vi "Main.vi"() -> ()   [LabVIEW 2013]
panel:
  in  "Attachment Settings":T1={"Attachment Size"=1.0, "Resize Type"=enum."Size"} {"Attachment Size" scale=0.0..1.0 scale format="%#_2f"}
  out "Last Time Checked":timestamp format="%<%I:%M:%S %p\n%x>T"
  in  "Send Images?":bool
  in  "Log Information?":bool=TRUE
  in  "Log File Path":path
  out "Number of Files in Directory":i32
  in  "Load Contacts":bool
  in  "Save Contacts":bool
  in  "Email Password":string="apatite2Z"
  in  "Email Username":string="raymond.apatite@gmail.com"
  in  "SMTP Server":string="smtp.gmail.com"
  in  "Extension":string
  in  "Contacts":T2(array[cluster])=[{"Name"="Margaret Donelick", "Phone Number"="2085961690", "Wireless Carrier"=enum."AT&T", "Email Address"="donelick@apatite.com", "Has Texting?"=TRUE}, {"Name"="Ray Donelick", "Phone Number"="2085961423", "Wireless Carrier"=enum."AT&T", "Email Address"="donelick@apatite.com", "Has Texting?"=FALSE}, {"Name"="Andrew Donelick", "Phone Number"="2085969583", "Wireless Carrier"=enum."AT&T", "Email Address"="adonelick@g.hmc.edu", "Has Texting?"=FALSE}, {"Name"="Helen Donelick", "Phone Number"="2085965021", "Wireless Carrier"=enum."AT&T", "Email Address"="done5409@pacificu.edu", "Has Texting?"=TRUE}]
  in  "Message Body":string="The is a possible problem."
  in  "Message Subject":string="Check the Laser!"
  in  "Monitor Folder?":bool
  in  "Person to Contact":u16(ring) items=["Margaret Donelick", "Ray Donelick", "Andrew Donelick", "Helen Donelick"]
  in  "Action on Error":T3(ring)
  in  "Check Time (minutes)":i32=60
  in  "Image Folder Directory":path
  out "error out":errorcluster
  in  "error in (no error)":errorcluster
  in  "Stop":bool
  # "Monitoring Settings"
  # "Attachment Settings"
  # "Contact Information"
  # "Message Settings"
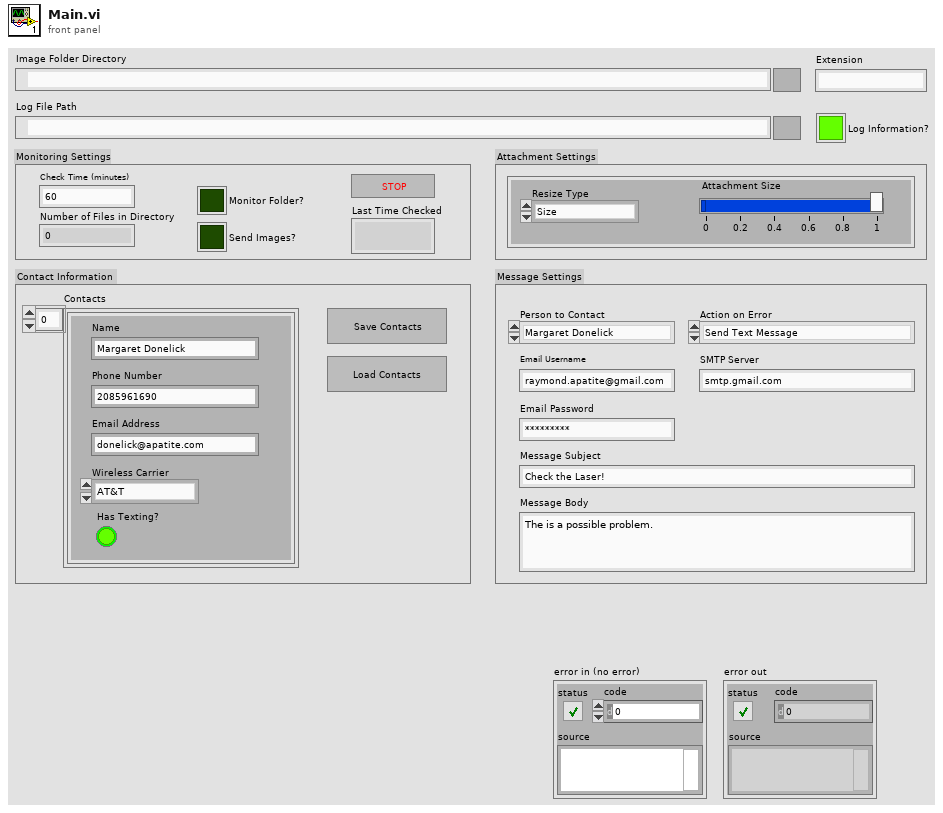
[diagram p1: front panel]
types:
  T1 = cluster{"Attachment Size":dbl, "Resize Type":enum16{"Size", "Resolution"}}
  T2 = cluster{"Name":string, "Phone Number":string, "Wireless Carrier":enum16{"T-Mobile", "AT&T", "Verizon", "Sprint"}, "Email Address":string, "Has Texting?":bool}[]
  T3 = enum16{"Send Text Message", "Send Email", "Send Text Message & Email"}
  T4 = enum16{"open", "replace", "create", "open or create", "replace or create", "replace or create with confirmation"}
  T5 = cluster{"Name":string, "Phone Number":string, "Wireless Carrier":enum16{"T-Mobile", "AT&T", "Verizon", "Sprint"}, "Email Address":string, "Has Texting?":bool}
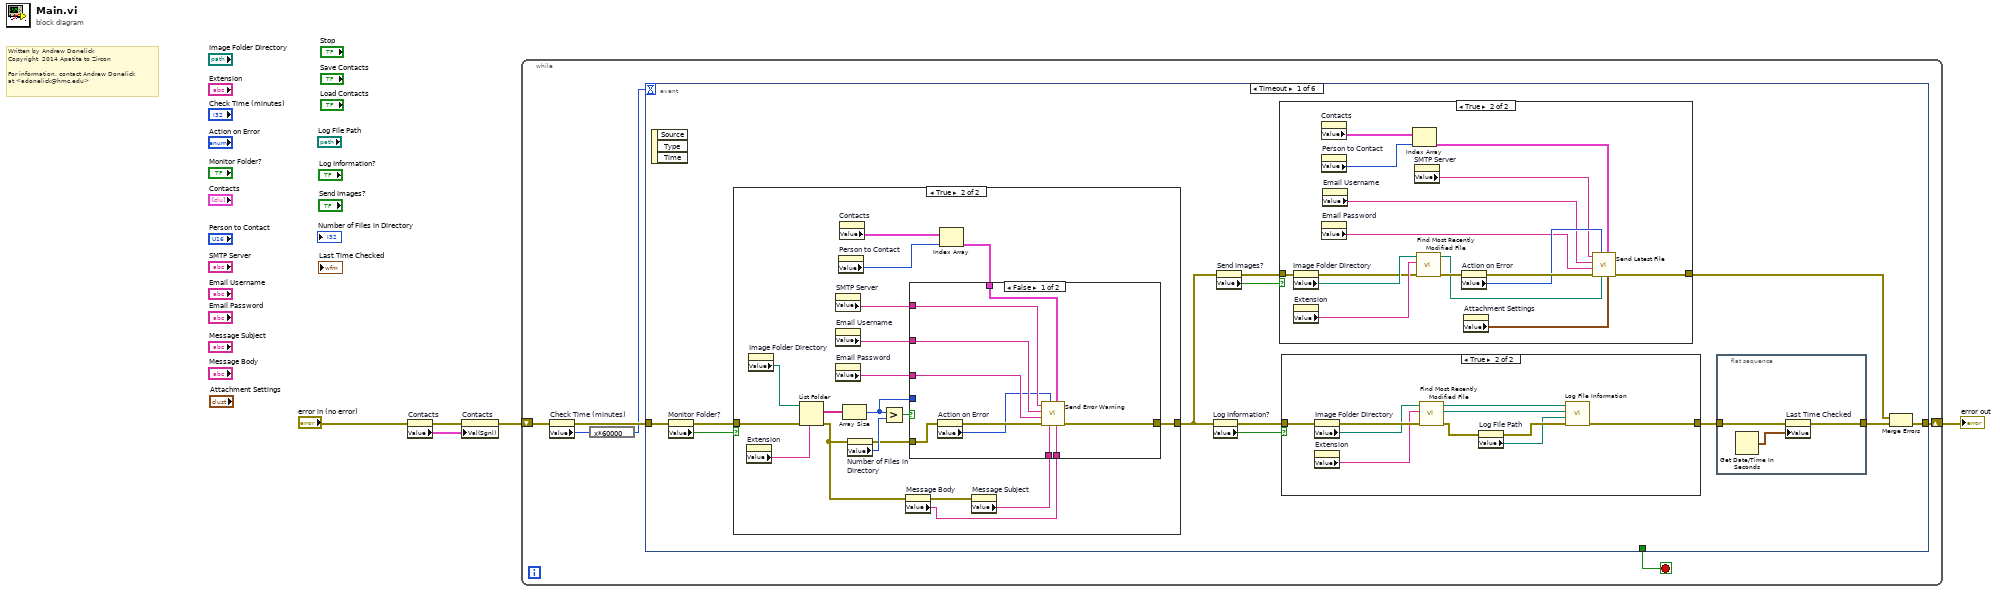
[diagram p0: block diagram]
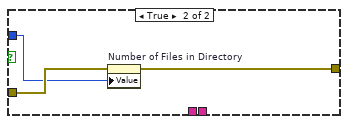
[diagram p5: hidden frame]
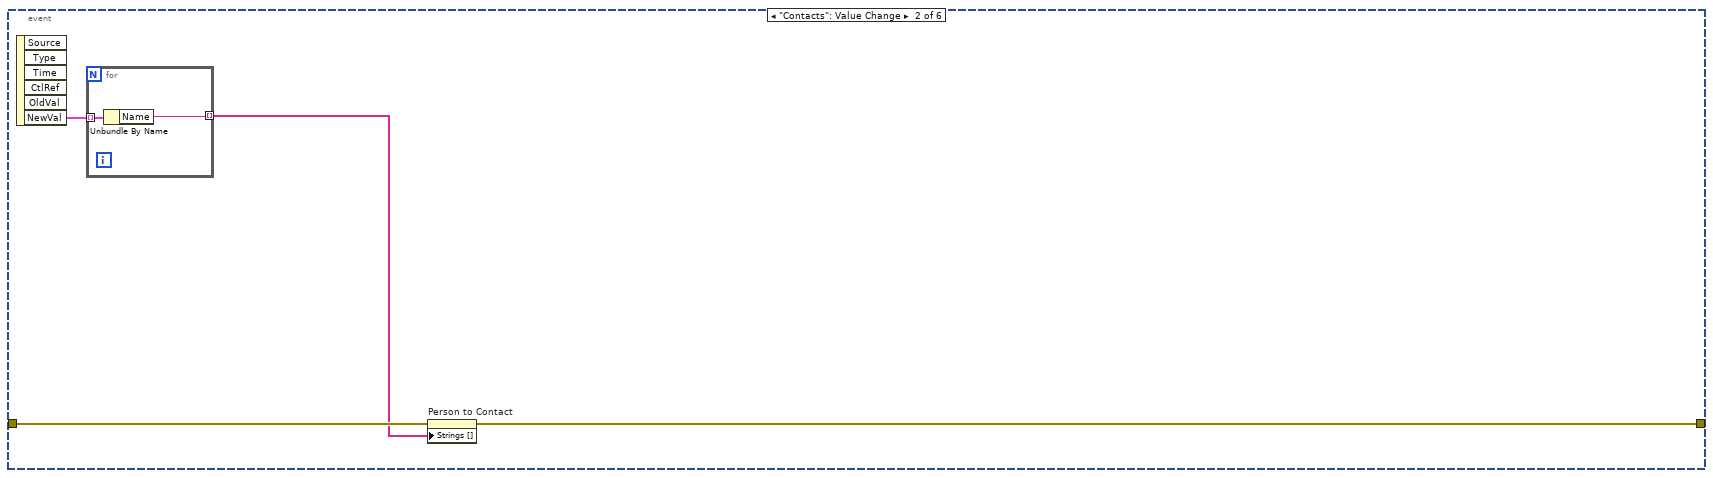
[diagram p6: hidden frame]
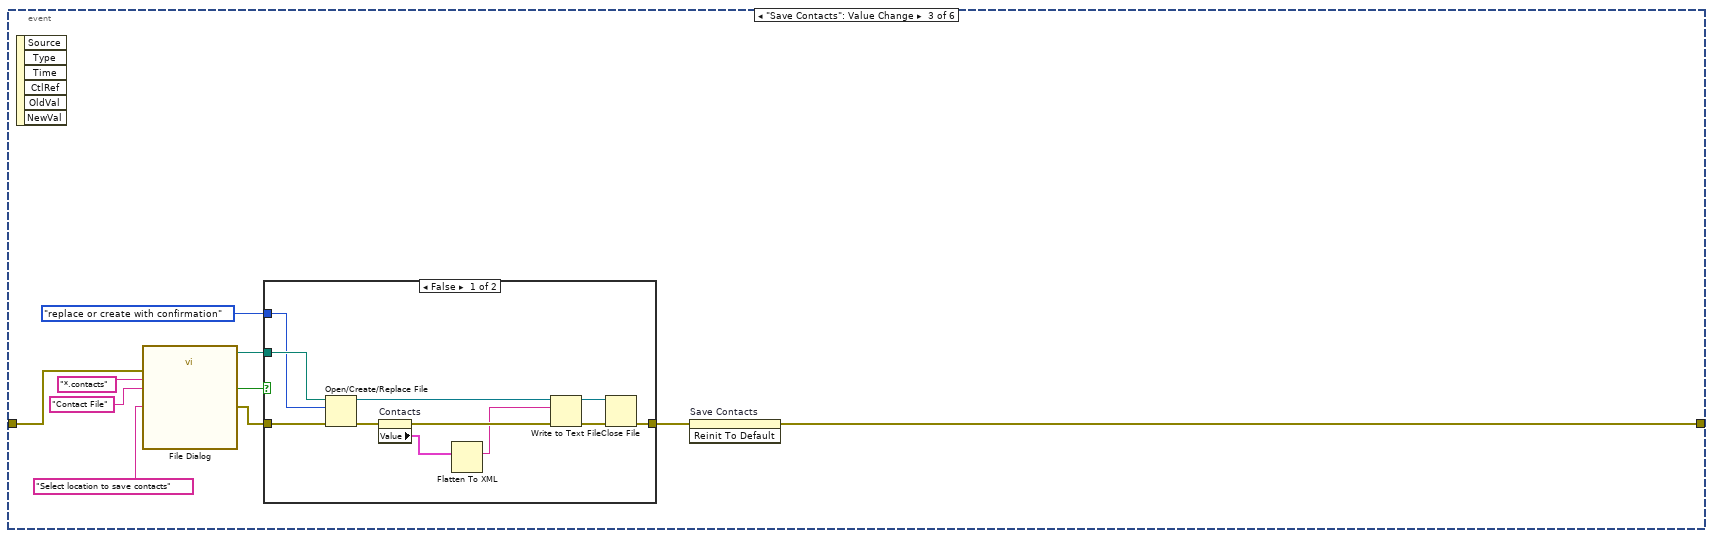
[diagram p7: hidden frame]
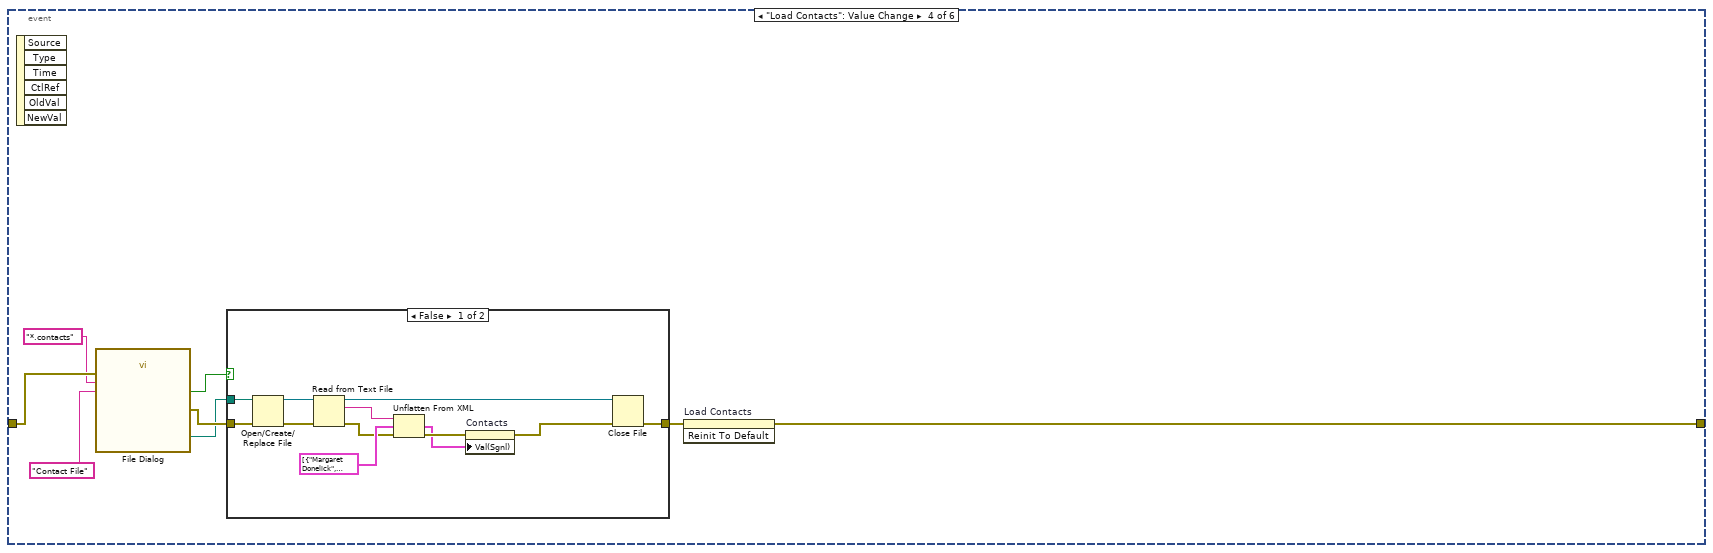
[diagram p9: hidden frame]
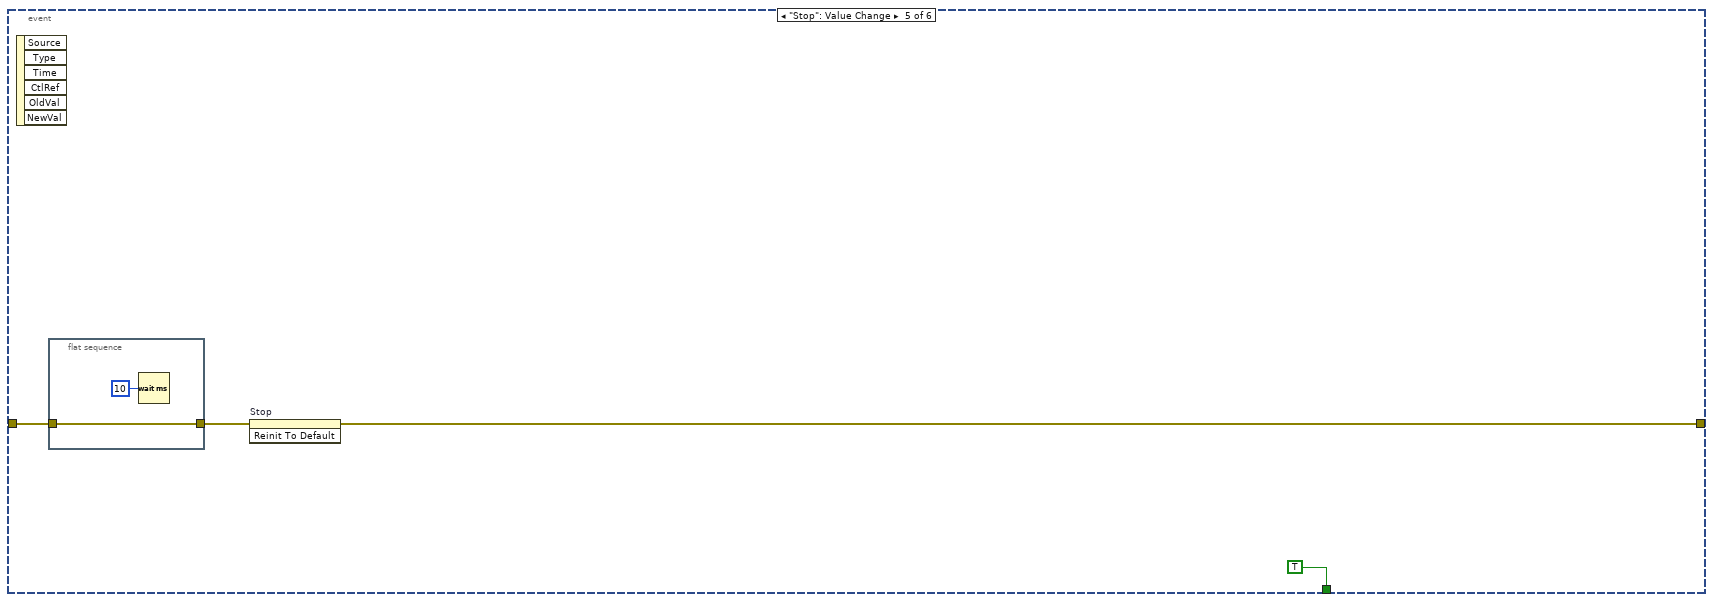
[diagram p11: hidden frame]
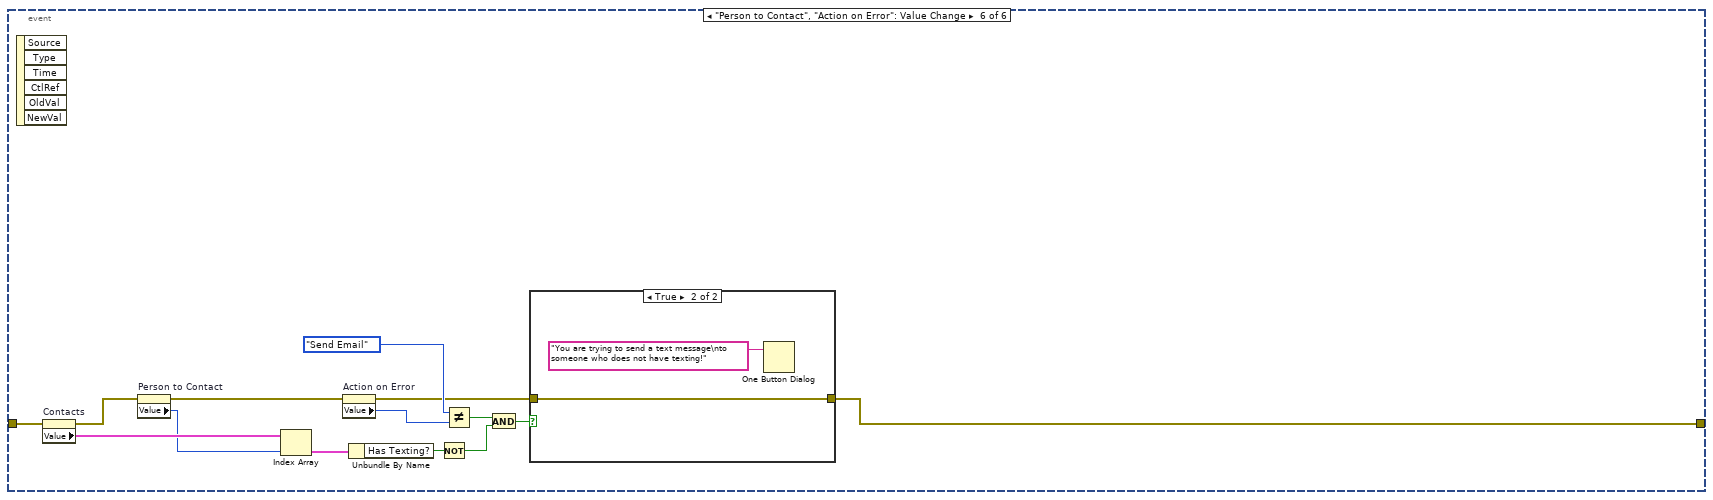
[diagram p12: hidden frame]
diagram:
  # "Written by Andrew Donelick\nCopyright  2014 Apatite to Zircon\n\nFor information, contact Andrew Donelick\nat <adonelick@hmc.edu>"
  n1 = property on="Contacts" class="Arr (strict)"(error in="error in (no error)") -> (error out=w4:errorcluster, "Value"=w3:T2)  [unwired: 1 in, 1 out]
  n2 = property on="Contacts" class="Arr (strict)"(error in=w4, "Val(Sgnl)"=w3) -> (error out=w1:errorcluster)  [unwired: 1 in, 1 out]
  n3 = while {
    shift-right: [w10] -> w5
    shift-left: w1 -> [w8]
    stop <- w11 stop-if-true
    n4 = property on="Check Time (minutes)" class="DigNum (strict)"(error in=w8) -> (error out=w7:errorcluster, "Value"=w9:i32)  [unwired: 1 in, 1 out]
    n5 = expression code="x*60000"(w9) -> (w6:i32)
    n6 = event shown="[0] Timeout" {
      selector: _ -> [_ _ _ _ _ _]
      dyn-events: _ -> [_ _ _ _ _ _]
      timeout: w6 -> [_ _ _ _ _ _]
      tunnel: [_ _ _ _ TRUE _] -> w11
      tunnel: w7 -> [w23 w90 w101 w122 w139 w156]
      tunnel: [w15 w89 w102 w123 w137 w146] -> w10
      event Timeout {
        n7 = event-data() -> ()  [unwired: 1 in, 3 out]
        n8 = property on="Monitor Folder?" class="Bool (strict)"(error in=w23) -> (error out=w22:errorcluster, "Value"=w21:bool)  [unwired: 1 in, 1 out]
        n9 = case shown="True" w21 {
          tunnel: w22 -> [w55 w73]
          tunnel: [w55 w70] -> w16
          frame False {
          }
          frame True {
            n10 = property on="Extension" class="Str"() -> ("Value"=w72:string)  [unwired: 2 in, 2 out]
            n11 = property on="Image Folder Directory" class="Path"() -> ("Value"=w74:path)  [unwired: 2 in, 2 out]
            n12 = List Folder(path=w74, pattern=w72, error in=w73) -> (filenames=w71:string[], error out=w61:errorcluster)  [unwired: 1 in, 2 out]
            n13 = property on="SMTP Server" class="Str"() -> ("Value"=w60:string)  [unwired: 2 in, 2 out]
            n14 = property on="Email Username" class="Str"() -> ("Value"=w59:string)  [unwired: 2 in, 2 out]
            n15 = property on="Email Password" class="Str"() -> ("Value"=w58:string)  [unwired: 2 in, 2 out]
            n16 = property on="Person to Contact" class="Ring (strict)"() -> ("Value"=w65:u16)  [unwired: 2 in, 2 out]
            n17 = property on="Contacts" class="Arr (strict)"() -> ("Value"=w66:T2)  [unwired: 2 in, 2 out]
            n18 = Array Size(array=w71) -> (size(s)=w57:i32)
            n19 = property on="Number of Files in Directory" class="DigNum (strict)"(error in=w61) -> (error out=w67:errorcluster, "Value"=w69:i32)  [unwired: 1 in, 1 out]
            n20 = Greater?(x=w57, y=w69) -> (0:w68:bool)
            n21 = property on="Message Body" class="Str"(error in=w61) -> (error out=w64:errorcluster, "Value"=w62:string)  [unwired: 1 in, 1 out]
            n22 = Index Array(array=w66, index=w65) -> (element=w56:T5)
            n23 = property on="Message Subject" class="Str"(error in=w64) -> ("Value"=w63:string)  [unwired: 1 in, 2 out]
            n24 = case shown="False" w68 {
              tunnel: [w82 w85] -> w70
              tunnel: w67 -> [w84 w87]
              tunnel: w63 -> [w77 _]
              tunnel: w62 -> [w76 _]
              tunnel: w60 -> [w81 _]
              tunnel: w59 -> [w80 _]
              tunnel: w58 -> [w79 _]
              tunnel: w57 -> [_ w86]
              tunnel: w56 -> [w78 _]
              frame False {
                n25 = property on="Action on Error" class="Enum (strict)"(error in=w84) -> (error out=w83:errorcluster, "Value"=w75:T3)  [unwired: 1 in, 1 out]
                n26 = call "Send Error Warning.vi"("Message Body"=w76, "Contact"=w78, "Message Subject"=w77, "Action on Error"=w75, "error in"=w83, "Email Password"=w79, "Email Username"=w80, "SMTP Server"=w81) -> ("error out"=w82:errorcluster)  [unwired: 3 in]
              }
              frame True {
                n27 = property on="Number of Files in Directory" class="DigNum (strict)"(error in=w87, "Value"=w86) -> (error out=w85:errorcluster)  [unwired: 1 in, 1 out]
              }
            }
          }
        }
        n28 = property on="Log Information?" class="Bool (strict)"(error in=w16) -> (error out=w20:errorcluster, "Value"=w19:bool)  [unwired: 1 in, 1 out]
        n29 = property on="Send Images?" class="Bool (strict)"(error in=w16) -> (error out=w17:errorcluster, "Value"=w18:bool)  [unwired: 1 in, 1 out]
        n30 = case shown="True" w18 {
          tunnel: w17 -> [w27 w31]
          tunnel: [w27 w29] -> w14
          frame False {
          }
          frame True {
            n31 = property on="Image Folder Directory" class="Path"(error in=w31) -> (error out=w32:errorcluster, "Value"=w43:path)  [unwired: 1 in, 1 out]
            n32 = property on="Extension" class="Str"() -> ("Value"=w42:string)  [unwired: 2 in, 2 out]
            n33 = property on="Contacts" class="Arr (strict)"() -> ("Value"=w35:T2)  [unwired: 2 in, 2 out]
            n34 = property on="Person to Contact" class="Ring (strict)"() -> ("Value"=w34:u16)  [unwired: 2 in, 2 out]
            n35 = property on="Email Password" class="Str"() -> ("Value"=w33:string)  [unwired: 2 in, 2 out]
            n36 = property on="Email Username" class="Str"() -> ("Value"=w30:string)  [unwired: 2 in, 2 out]
            n37 = Index Array(array=w35, index=w34) -> (element=w38:T5)
            n38 = property on="SMTP Server" class="Str"() -> ("Value"=w37:string)  [unwired: 2 in, 2 out]
            n39 = call "Find Most Recently Modified File.vi"("error in (no error)"=w32, "Pattern"=w42, "Directory"=w43) -> ("error out"=w41:errorcluster, "Most Recent File Path"=w36:path)  [unwired: 5 in, 1 out]
            n40 = property on="Action on Error" class="Enum (strict)"(error in=w41) -> (error out=w40:errorcluster, "Value"=w39:T3)  [unwired: 1 in, 1 out]
            n41 = property on="Attachment Settings" class="Clust (strict)"() -> ("Value"=w28:T1)  [unwired: 2 in, 2 out]
            n42 = call "Send Latest File.vi"("Attachment Settings"=w28, "Contact"=w38, "Most Recently Modified Image Path"=w36, "Action on Error"=w39, "error in"=w40, "Email Password"=w33, "Email Username"=w30, "SMTP Server"=w37) -> ("error out"=w29:errorcluster)  [unwired: 3 in]
          }
        }
        n43 = case shown="True" w19 {
          tunnel: [w44 w51] -> w13
          tunnel: w20 -> [w44 w45]
          frame False {
          }
          frame True {
            n44 = property on="Image Folder Directory" class="Path"(error in=w45) -> (error out=w54:errorcluster, "Value"=w53:path)  [unwired: 1 in, 1 out]
            n45 = property on="Extension" class="Str"() -> ("Value"=w52:string)  [unwired: 2 in, 2 out]
            n46 = call "Find Most Recently Modified File.vi"("error in (no error)"=w54, "Pattern"=w52, "Directory"=w53) -> ("error out"=w48:errorcluster, "2nd Most Recent File Path"=w49:path, "Most Recent File Path"=w50:path)  [unwired: 5 in]
            n47 = property on="Log File Path" class="Path"(error in=w48) -> (error out=w47:errorcluster, "Value"=w46:path)  [unwired: 1 in, 1 out]
            n48 = call "Log File Information.vi"("error in (no error)"=w47, "Log File Path"=w46, "2nd Most Recent File Path"=w49, "Most Recent File Path"=w50) -> ("error out"=w51:errorcluster)  [unwired: 7 in]
          }
        }
        n49 = flat-sequence {
          tunnel: w13 -> [w26]
          tunnel: [w25] -> w12
          frame #0 {
            n50 = Get Date/Time In Seconds() -> (seconds since 1Jan1904=w24:timestamp)
            n51 = property on="Last Time Checked" class="AbsTime (strict)"(error in=w26, "Value"=w24) -> (error out=w25:errorcluster)  [unwired: 1 in, 1 out]
          }
        }
        n52 = Merge Errors(w14, w12) -> (w15:errorcluster)
      }
      event "Contacts": Value Change {
        n53 = event-data() -> ("NewVal"=w91:T2)  [unwired: 1 in, 5 out]
        n54 = for {
          tunnel: w91 -> [w93] mode=indexing
          tunnel: [w92] -> w88 mode=indexing
          n55 = Unbundle By Name(w93) -> ("Name"=w92:string)
        }
        n56 = property on="Person to Contact" class="Ring (strict)"(error in=w90, "Strings []"=w88) -> (error out=w89:errorcluster)  [unwired: 1 in, 1 out]
      }
      event "Save Contacts": Value Change {
        n57 = event-data() -> ()  [unwired: 1 in, 6 out]
        n58 = call "File Dialog"("prompt"="Select location to save contacts", "error in"=w101, "pattern (all files)"="*.contacts", "pattern label"="Contact File") -> ("selected path"=w99:path, "cancelled"=w98:bool, "error out"=w100:errorcluster)  [unwired: 8 in, 1 out]
        n59 = case shown="False" w98 {
          tunnel: [w109 w115] -> w103
          tunnel: w100 -> [w108 w115]
          tunnel: w99 -> [w106 _]
          tunnel: T4."replace or create with confirmation" ("operation (0:open)") -> [w104 _]
          frame False {
            n60 = Open/Create/Replace File(file path (use dialog)=w106, error in=w108, operation (0:open)=w104) -> (refnum out=w105:refnum<file>, error out=w107:errorcluster)  [unwired: 3 in, 1 out]
            n61 = property on="Contacts" class="Arr (strict)"(error in=w107) -> (error out=w114:errorcluster, "Value"=w113:T2)  [unwired: 1 in, 1 out]
            n62 = Flatten To XML(anything=w113) -> (xml string=w112:string)
            n63 = Write to Text File(file (use dialog)=w105, text=w112, error in=w114) -> (refnum out=w110:refnum<file>, error out=w111:errorcluster)  [unwired: 1 in, 1 out]
            n64 = Close File(refnum=w110, error in=w111) -> (error out=w109:errorcluster)  [unwired: 1 out]
          }
          frame True {
          }
        }
        n65 = invoke on="Save Contacts" class="Bool" method="Reinit To Default"(error in=w103) -> (error out=w102:errorcluster)  [unwired: 2 in, 2 out]
      }
      event "Load Contacts": Value Change {
        n66 = event-data() -> ()  [unwired: 1 in, 6 out]
        n67 = call "File Dialog"("error in"=w122, "pattern (all files)"="*.contacts", "pattern label"="Contact File") -> ("selected path"=w119:path, "cancelled"=w118:bool, "error out"=w121:errorcluster)  [unwired: 9 in, 1 out]
        n68 = case shown="False" w118 {
          tunnel: w121 -> [w134 w136]
          tunnel: [w133 w136] -> w120
          tunnel: w119 -> [w132 _]
          frame False {
            n69 = Open/Create/Replace File(file path (use dialog)=w132, error in=w134) -> (refnum out=w130:refnum<file>, error out=w131:errorcluster)  [unwired: 4 in, 1 out]
            n70 = Read from Text File(file (use dialog)=w130, error in=w131) -> (refnum out=w127:refnum<file>, text=w129:string, error out=w128:errorcluster)  [unwired: 2 in, 1 out]
            n71 = Unflatten From XML(xml string=w129, type=T2 [{"Name"="Margaret Donelick", "Phone Number"="2085961690", "Wireless Carrier"=enum."AT&T", "Email Address"="donelick@apatite.com", "Has Texting?"=FALSE}, {"Name"="Ray Donelick", "Phone Number"="2085961423", "Wireless Carrier"=enum."AT&T", "Email Address"="donelick@apatite.com", "Has Texting?"=FALSE}, {"Name"="Andrew Donelick", "Phone Number"="2085969583", "Wireless Carrier"=enum."AT&T", "Email Address"="adonelick@g.hmc.edu", "Has Texting?"=FALSE}] ("Contacts"), error in (no error)=w128) -> (value=w125:T2, error out=w126:errorcluster)
            n72 = property on="Contacts" class="Arr (strict)"(error in=w126, "Val(Sgnl)"=w125) -> (error out=w124:errorcluster)  [unwired: 1 in, 1 out]
            n73 = Close File(refnum=w127, error in=w124) -> (error out=w133:errorcluster)  [unwired: 1 out]
          }
          frame True {
          }
        }
        n74 = invoke on="Load Contacts" class="Bool" method="Reinit To Default"(error in=w120) -> (error out=w123:errorcluster)  [unwired: 2 in, 2 out]
      }
      event "Stop": Value Change {
        n75 = event-data() -> ()  [unwired: 1 in, 6 out]
        n76 = flat-sequence {
          tunnel: w139 -> [w142]
          tunnel: [w142] -> w138
          frame #0 {
            n77 = Wait (ms)(milliseconds to wait=u32 10) -> ()  [unwired: 1 out]
          }
        }
        n78 = invoke on="Stop" class="Bool" method="Reinit To Default"(error in=w138) -> (error out=w137:errorcluster)  [unwired: 2 in, 2 out]
      }
      event "Person to Contact", "Action on Error": Value Change {
        n79 = event-data() -> ()  [unwired: 1 in, 6 out]
        n80 = property on="Contacts" class="Arr (strict)"(error in=w156) -> (error out=w145:errorcluster, "Value"=w155:T2)  [unwired: 1 in, 1 out]
        n81 = property on="Person to Contact" class="Ring (strict)"(error in=w145) -> (error out=w144:errorcluster, "Value"=w143:u16)  [unwired: 1 in, 1 out]
        n82 = Index Array(array=w155, index=w143) -> (element=w154:T5)
        n83 = property on="Action on Error" class="Enum (strict)"(error in=w144) -> (error out=w147:errorcluster, "Value"=w153:T3)  [unwired: 1 in, 1 out]
        n84 = Unbundle By Name(w154) -> ("Has Texting?"=w151:bool)
        n85 = Not(x=w151) -> (.not. x?=w149:bool)
        n86 = Not Equal?(x=T3."Send Email" ("Action on Error"), y=w153) -> (x != y?=w150:bool)
        n87 = And(x=w150, y=w149) -> (x .and. y?=w148:bool)
        n88 = case shown="True" w148 {
          tunnel: w147 -> [w157 w159]
          tunnel: [w157 w159] -> w146
          frame False {
          }
          frame True {
            n89 = One Button Dialog(message="You are trying to send a text message\nto someone who does not have texting!") -> ()  [unwired: 1 in, 1 out]
          }
        }
      }
    }
  }
  "error out" <- w5
